vi "Global 5.vi"() -> ()   [LabVIEW 2017]
panel:
  out "Count Encode":dbl
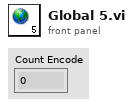
[diagram p1: front panel]
diagram:
